vi "DAQ_Manager.TestLauncher.vi"() -> ()   [LabVIEW 2016, in "DAQ_Manager.lvclass"]
uses:
  DAQ_Manager.lvclass
  <vilib>/JKI/JKI SMO/SMO/Typedefs/SMOState --Enum.ctl
  C:/Program Files (x86)/National Instruments/LabVIEW 2016/vi.lib/JKI/JKI SMO/SMO/SMO.lvclass
  <vilib>/JKI/JKI SMO/SMO/SMO.lvclass
panel:
  out "getWaveforms":waveform(dbl)[](graph)
  out "SMO State":T1
  out "error out":errorcluster
  in  "Stop":bool
  # "DAQ Manager SMO Test Launcher"
  # "For instructions on how to use the JKI State Machine Objects, examples and video tutorials, visit:\nhttp://jki.net/state-machine-objects/\n\nJKI State Machine Objects™\nhttp://jki.net/state-machine-objects/\nCopyright (C) 2005-2015, JKI <info@jki.net>\nALL RIGHTS RESERVED"
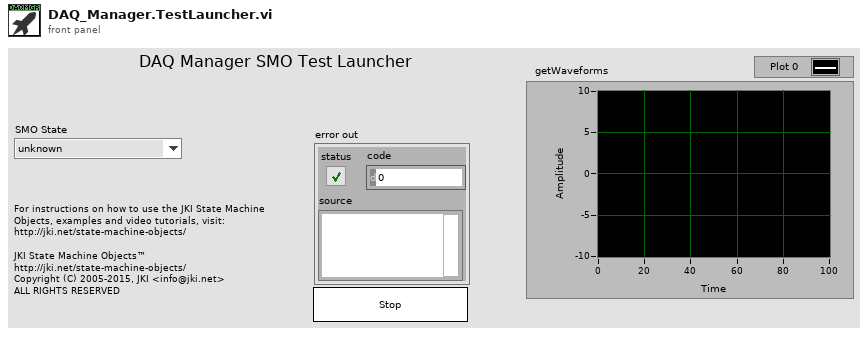
[diagram p1: front panel]
types:
  T1 = typedef "SMO.lvclass/SMOState --Enum.ctl" = enum16{"unknown", "Created", "Started", "Stopped"}
  T2 = typedef "SMO.lvclass/Public Events.ctl" = cluster{"Error":refnum<user-event>, "State":refnum<user-event>, "Reserve State":refnum<user-event>}
  T3 = typedef "DAQ_Manager.lvclass/PublicEvents--Cluster.ctl" = cluster{"getWaveform":refnum<user-event>}
  T4 = cluster{"Event Registration Refnum":refnum<event-registration>}
  T5 = typedef "DAQ_Manager.lvclass/PublicEvents--DAQ_Manager.getWaveform.ctl" = waveform(dbl)[]
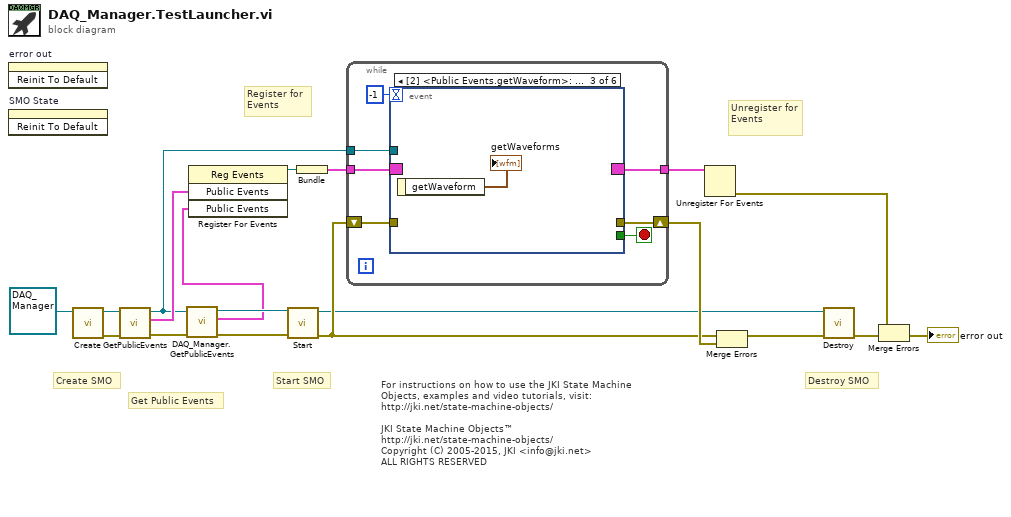
[diagram p0: block diagram]
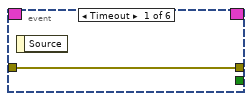
[diagram p2: hidden frame]
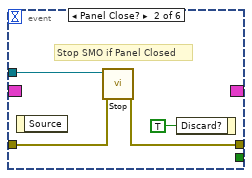
[diagram p3: hidden frame]
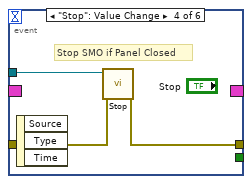
[diagram p4: hidden frame]
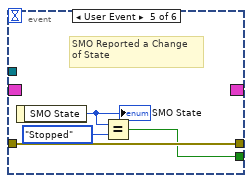
[diagram p5: hidden frame]
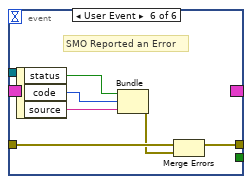
[diagram p6: hidden frame]
diagram:
  # "For instructions on how to use the JKI State Machine Objects, examples and video tutorials, visit:\nhttp://jki.net/state-machine-objects/\n\nJKI State Machine Objects™\nhttp://jki.net/state-machine-objects/\nCopyright (C) 2005-2015, JKI <info@jki.net>\nALL RIGHTS RESERVED"
  # "Get Public Events"
  # "Start SMO"
  # "Destroy SMO"
  # "Create SMO"
  # "Unregister for Events"
  # "Register for Events"
  n1 = invoke on="error out" class="Clust (strict)" method="Reinit To Default"() -> ()  [unwired: 3 in, 3 out]
  n2 = invoke on="SMO State" class="Enum (strict)" method="Reinit To Default"() -> ()  [unwired: 3 in, 3 out]
  n3 = call <vilib>:"Create.vi"("SMO"=refnum<class "DAQ_Manager.lvclass"> refnum ("SMO.Template.lvclass")) -> ("error out"=w8:errorcluster, "SMO out"=w9:refnum<class "DAQ_Manager.lvclass">)  [unwired: 8 in, 1 out]
  n4 = call <vilib>:"GetPublicEvents.vi"("error in (no error)"=w8, "SMO"=w9) -> ("error out"=w5:errorcluster, "Public Events"=w7:T2, "SMO out"=w4:refnum<class "DAQ_Manager.lvclass">)  [unwired: 7 in]
  n5 = call "DAQ_Manager.GetPublicEvents.vi"("error in (no error)"=w5, "DAQ_Manager"=w4) -> ("error out"=w3:errorcluster, "Public Events"=w1:T3, "DAQ_Manager out"=w2:refnum<class "DAQ_Manager.lvclass">)  [unwired: 7 in]
  n6 = register-events(w7, w1) -> (reference out=w6:refnum<event-registration>)  [unwired: 2 in, 1 out]
  n7 = call <vilib>:"Start.vi"("error in (no error)"=w3, "SMO"=w2) -> ("error out"=w12:errorcluster, "SMO out"=w10:refnum<class "DAQ_Manager.lvclass">)  [unwired: 8 in]
  n8 = Bundle("Event Registration Refnum"=w6) -> (w18:T4)  [unwired: 1 in]
  n9 = while {
    shift-right: [w25] -> w17
    shift-left: w12 -> [w24]
    tunnel: w18 -> [w23]
    tunnel: [w22] -> w19
    tunnel: w4 -> [w21]
    stop <- w26 stop-if-true
    n10 = event shown="[2] <Public Events.getWaveform>: User Event" {
      selector: w23 -> [_ _ _ _ _ _]
      dyn-events: [_ _ _ _ _ _] -> w22
      timeout: -1 -> [_ _ _ _ _ _]
      tunnel: [_ _ _ _ w36 _] -> w26
      tunnel: w21 -> [_ w31 _ w35 _ _]
      tunnel: [w27 w30 _ w34 w39 w43] -> w25
      tunnel: w24 -> [w27 w29 _ w33 w39 w41]
      event Timeout {
        n11 = event-data() -> ()  [unwired: 1 in, 1 out]
      }
      event Panel Close? {
        # "Stop SMO if Panel Closed"
        n12 = event-data() -> ()  [unwired: 1 in, 1 out]
        n13 = call <vilib>:"Stop.vi"("error in (no error)"=w29, "SMO"=w31) -> ("error out"=w30:errorcluster)  [unwired: 8 in, 1 out]
        n14 = event-data("Discard?"=TRUE ("OK")) -> ()  [unwired: 1 in, 1 out]
      }
      event User Event {
        n15 = event-data() -> ("getWaveform"=→"getWaveforms":T5)  [unwired: 1 in]
      }
      event "Stop": Value Change {
        # "Stop SMO if Panel Closed"
        n16 = event-data() -> ()  [unwired: 1 in, 3 out]
        n17 = call <vilib>:"Stop.vi"("error in (no error)"=w33, "SMO"=w35) -> ("error out"=w34:errorcluster)  [unwired: 8 in, 1 out]
      }
      event User Event {
        # "SMO Reported a Change\nof State"
        n18 = event-data() -> ("SMO State"=w38:T1)  [unwired: 1 in]
        "SMO State" <- w38
        n19 = Equal?(x=w38, y=SMOState_--Enum."Stopped") -> (x = y?=w36:bool)
      }
      event User Event {
        # "SMO Reported an Error"
        n20 = event-data() -> ("status"=w42:bool, "code"=w45:i32, "source"=w44:string)  [unwired: 1 in]
        n21 = Bundle("status"=w42, "code"=w45, "source"=w44) -> (w40:errorcluster)  [unwired: 1 in]
        n22 = Merge Errors(w41, w40) -> (w43:errorcluster)
      }
    }
  }
  n23 = Unregister For Events(event registration refnum=w19) -> (error out=w16:errorcluster)  [unwired: 1 in]
  n24 = Merge Errors(w12, w17) -> (w11:errorcluster)
  n25 = call <vilib>:"Destroy.vi"("error in (no error)"=w11, "SMO"=w10) -> ("error out"=w14:errorcluster)  [unwired: 9 in]
  n26 = Merge Errors(w16, w14) -> (→"error out":errorcluster)
